vi "Endpoint Connected.vi"(8 "error in":errorcluster, 10 "Endpoint":refnum<class "Message Enqueuer.lvclass">, 11 "Host Reply Time Test Actor in":refnum<class "Host Reply Time Test Actor.lvclass">) -> (0 "error out":errorcluster, 3 "Host Reply Time Test Actor out":refnum<class "Host Reply Time Test Actor.lvclass">)   [LabVIEW 2023, in "Host Reply Time Test Actor.lvlib" / "Host Reply Time Test Actor.lvclass"]
doc: "Override this method to specify how the receiving actor responds to a Connected message from a nested endpoint actor."
uses:
  Host Reply Time Test Actor.lvclass
  <vilib>/ActorFramework/Message Enqueuer/Message Enqueuer.lvclass
  Host Reply Time Test Actor.lvclass/Host Reply Time Test Actor.ctl
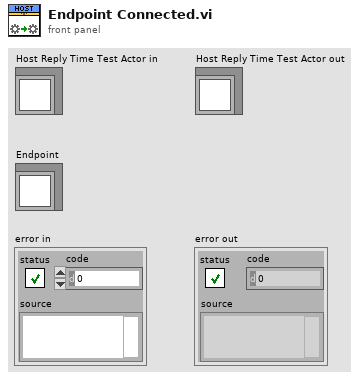
[diagram p1: front panel]
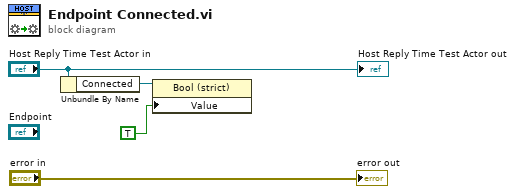
[diagram p0: block diagram]
diagram:
  n1 = Unbundle By Name("Host Reply Time Test Actor in") -> ("Connected"=w3:refnum<vi>)
  n2 = property class="Bool (strict)"(reference=w3, "Value"=TRUE) -> ()  [unwired: 1 in, 2 out]
  "error out" <- "error in"
  "Host Reply Time Test Actor out" <- "Host Reply Time Test Actor in"
